vi "Fc_update_params_from_uc.vi"(7 "Class TCP":T1, 8 "error in (no error)":errorcluster, 9 "Trace names":refnum<vi>, 10 "# Control":refnum<vi>, 11 "SamplesXSignal?":refnum<vi>) -> (0 "error out":errorcluster, 1 "TRACE_SIZE":i32, 2 "NB_TRACED_SIGNALS":i32, 3 "CS STATUS":i32)   [LabVIEW 2022 SP3]
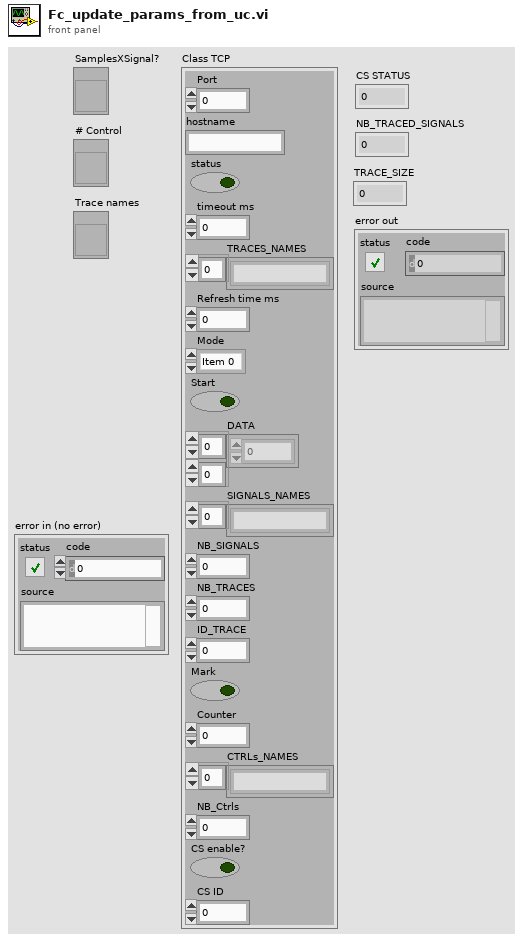
[diagram p1: front panel]
types:
  T1 = cluster{"Port":i32, "hostname":string, "status":bool, "timeout ms":i32, "TRACES_NAMES":string[], "Refresh time ms":i32, "Mode":enum32{"Item 0", "Item 1"}, "Start":bool, "DATA":sgl[][], "SIGNALS_NAMES":string[], "NB_SIGNALS":i32, "NB_TRACES":i32, "ID_TRACE":i32, "Mark":bool, "Counter":i32, "CTRLs_NAMES":string[], "NB_Ctrls":i32, "CS enable?":bool, "CS ID":i32}
  T2 = cluster{"TRACE_SIZE":i32, "CS_ID":i32, "TRACE ID":i32, "CMD":i32, "DATA(M)":i32}
  T3 = cluster{"timeout ms":i32, "remote port":u16, "Address":string}
  T4 = cluster{"SIZE":i32, " TRACE DATA":sgl[], "TRACE_SIZE":i32, "NB_TRACES":i32, "NB_TRACED_SIGNALS":i32, "NAMES TRACED SIGNALS":string[], "NAMES TRACES":string[], "CS STATUS":i32, "NB_CSs":i32, "NAMES CSs":string[], "DATA (M)":sgl[], "CMD":i32}
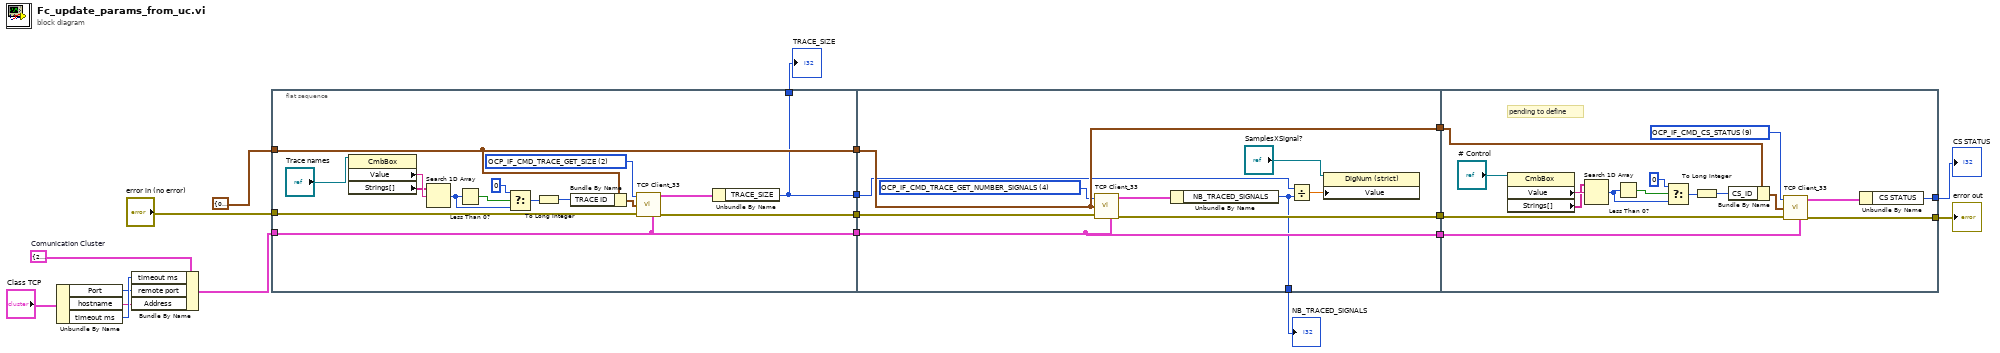
[diagram p0: block diagram]
diagram:
  w12 = T3 {"timeout ms"=2000, "remote port"=8085, "Address"="127.0.0.1"}  # Comunication Cluster
  n1 = Unbundle By Name("Class TCP") -> ("Port"=w3:i32, "hostname"=w4:string, "timeout ms"=w5:i32)
  n2 = Bundle By Name(cluster=w12, "timeout ms"=w5, "remote port"=w3, "Address"=w4) -> (w6:T3)
  n3 = flat-sequence {
    tunnel: T2 {"TRACE_SIZE"=0, "CS_ID"=0, "TRACE ID"=0, "CMD"=0, "DATA(M)"=0} ("Input Cluster") -> [w32]
    tunnel: [w32] -> w19
    tunnel: [w34] -> w18
    tunnel: w6 -> [w33]
    tunnel: [w33] -> w17
    tunnel: [w24] -> w16
    tunnel: [w24] -> w9
    tunnel: "error in (no error)" -> [w20]
    tunnel: w19 -> [w43]
    tunnel: [w43] -> w15
    tunnel: w18 -> [w45]
    tunnel: [w44] -> w14
    tunnel: w17 -> [w42]
    tunnel: [w42] -> w13
    tunnel: w16 -> [w39]
    tunnel: [w38] -> w10
    tunnel: [w57] -> w2
    tunnel: w15 -> [w60]
    tunnel: w14 -> [w56]
    tunnel: w13 -> [w55]
    tunnel: [w49] -> w11
    frame #0 {
      w35 = 2 items=["OCP_IF_CMD_TRACE_READ", "OCP_IF_CMD_TRACE_RESET", "OCP_IF_CMD_TRACE_GET_SIZE", "OCP_IF_CMD_TRACE_SET_SIZE", "OCP_IF_CMD_TRACE_GET_NUMBER_SIGNALS", "OCP_IF_CMD_TRACE_GET_SIGNALS_NAMES", "OCP_IF_CMD_TRACE_GET_NUMBER_TRACES", "OCP_IF_CMD_TRACE_GET_TRACES_NAMES", "OCP_IF_CMD_TRACE_GET_ADDRESS", "OCP_IF_CMD_CS_STATUS", "OCP_IF_CMD_CS_ENABLE", "OCP_IF_CMD_CS_DISABLE", "OCP_IF_CMD_CS_CONTROLLER_IF", "OCP_IF_CMD_CS_HARDWARE_IF", "OCP_IF_CMD_CS_GET_NUMBER_CONTROLLERS", "OCP_IF_CMD_CS_GET_CONTROLLERS_NAMES", "OCP_IF_CMD_PLATFORM_ID", "OCP_IF_CMD_PLATFORM_IF", "OCP_IF_CMD_OPIL_UPDATE_MEASUREMENTS", "OCP_IF_CMD_OPIL_UPDATE_SIM_DATA", "OCP_IF_CMD_OPIL_RUN_CONTROL", "OCP_IF_CMD_OPIL_INITIALIZE_CONTROL", "OCP_IF_CMD_OPIL_GET_CONTROL", "OCP_IF_CMD_OPIL_GET_CONTROLLER_DATA", "OCP_IF_CMD_END"] ("CMD")
      n4 = property class="CmbBox"(reference="Trace names") -> ("Value"=w23:string, "Strings[]"=w22:string[])  [unwired: 1 in, 2 out]
      n5 = Search 1D Array(1D array=w22, element=w23) -> (index of element=w26:i32)  [unwired: 1 in]
      n6 = Less Than 0?(x=w26) -> (x < 0?=w27:bool)
      n7 = Select(t=0, s=w27, f=w26) -> (s? t:f=w25:i32)
      n8 = To Long Integer(number=w25) -> (32bit integer=w29:i32)
      n9 = Bundle By Name(cluster=w32, "TRACE ID"=w29) -> (w31:T2)
      n10 = call "TCP Client_33.vi"("CMD"=w35, "Input Cluster"=w31, "error in (no error)"=w20, "Comunication Cluster"=w33) -> ("Output cluster"=w30:T4, "error out"=w34:errorcluster)  [unwired: 4 in, 1 out]
      n11 = Unbundle By Name(w30) -> ("TRACE_SIZE"=w24:i32)
    }
    frame #1 {
      w41 = 4 items=["OCP_IF_CMD_TRACE_READ", "OCP_IF_CMD_TRACE_RESET", "OCP_IF_CMD_TRACE_GET_SIZE", "OCP_IF_CMD_TRACE_SET_SIZE", "OCP_IF_CMD_TRACE_GET_NUMBER_SIGNALS", "OCP_IF_CMD_TRACE_GET_SIGNALS_NAMES", "OCP_IF_CMD_TRACE_GET_NUMBER_TRACES", "OCP_IF_CMD_TRACE_GET_TRACES_NAMES", "OCP_IF_CMD_TRACE_GET_ADDRESS", "OCP_IF_CMD_CS_STATUS", "OCP_IF_CMD_CS_ENABLE", "OCP_IF_CMD_CS_DISABLE", "OCP_IF_CMD_CS_CONTROLLER_IF", "OCP_IF_CMD_CS_HARDWARE_IF", "OCP_IF_CMD_CS_GET_NUMBER_CONTROLLERS", "OCP_IF_CMD_CS_GET_CONTROLLERS_NAMES", "OCP_IF_CMD_PLATFORM_ID", "OCP_IF_CMD_PLATFORM_IF", "OCP_IF_CMD_OPIL_UPDATE_MEASUREMENTS", "OCP_IF_CMD_OPIL_UPDATE_SIM_DATA", "OCP_IF_CMD_OPIL_RUN_CONTROL", "OCP_IF_CMD_OPIL_INITIALIZE_CONTROL", "OCP_IF_CMD_OPIL_GET_CONTROL", "OCP_IF_CMD_OPIL_GET_CONTROLLER_DATA", "OCP_IF_CMD_END"] ("CMD")
      n12 = call "TCP Client_33.vi"("CMD"=w41, "Input Cluster"=w43, "error in (no error)"=w45, "Comunication Cluster"=w42) -> ("Output cluster"=w40:T4, "error out"=w44:errorcluster)  [unwired: 4 in, 1 out]
      n13 = Unbundle By Name(w40) -> ("NB_TRACED_SIGNALS"=w38:i32)
      n14 = Divide(x=w39, y=w38) -> (x/y=w37:dbl)
      n15 = property class="DigNum (strict)"(reference="SamplesXSignal?", "Value"=w37) -> ()  [unwired: 1 in, 2 out]
    }
    frame #2 {
      w59 = 9 items=["OCP_IF_CMD_TRACE_READ", "OCP_IF_CMD_TRACE_RESET", "OCP_IF_CMD_TRACE_GET_SIZE", "OCP_IF_CMD_TRACE_SET_SIZE", "OCP_IF_CMD_TRACE_GET_NUMBER_SIGNALS", "OCP_IF_CMD_TRACE_GET_SIGNALS_NAMES", "OCP_IF_CMD_TRACE_GET_NUMBER_TRACES", "OCP_IF_CMD_TRACE_GET_TRACES_NAMES", "OCP_IF_CMD_TRACE_GET_ADDRESS", "OCP_IF_CMD_CS_STATUS", "OCP_IF_CMD_CS_ENABLE", "OCP_IF_CMD_CS_DISABLE", "OCP_IF_CMD_CS_CONTROLLER_IF", "OCP_IF_CMD_CS_HARDWARE_IF", "OCP_IF_CMD_CS_GET_NUMBER_CONTROLLERS", "OCP_IF_CMD_CS_GET_CONTROLLERS_NAMES", "OCP_IF_CMD_PLATFORM_ID", "OCP_IF_CMD_PLATFORM_IF", "OCP_IF_CMD_OPIL_UPDATE_MEASUREMENTS", "OCP_IF_CMD_OPIL_UPDATE_SIM_DATA", "OCP_IF_CMD_OPIL_RUN_CONTROL", "OCP_IF_CMD_OPIL_INITIALIZE_CONTROL", "OCP_IF_CMD_OPIL_GET_CONTROL", "OCP_IF_CMD_OPIL_GET_CONTROLLER_DATA", "OCP_IF_CMD_END"] ("CMD")
      # "pending to define"
      n16 = property class="CmbBox"(reference="# Control") -> ("Value"=w48:string, "Strings[]"=w47:string[])  [unwired: 1 in, 2 out]
      n17 = Search 1D Array(1D array=w47, element=w48) -> (index of element=w52:i32)  [unwired: 1 in]
      n18 = Less Than 0?(x=w52) -> (x < 0?=w54:bool)
      n19 = Select(t=0, s=w54, f=w52) -> (s? t:f=w51:i32)
      n20 = To Long Integer(number=w51) -> (32bit integer=w50:i32)
      n21 = Bundle By Name(cluster=w60, "CS_ID"=w50) -> (w58:T2)
      n22 = call "TCP Client_33.vi"("CMD"=w59, "Input Cluster"=w58, "error in (no error)"=w56, "Comunication Cluster"=w55) -> ("Output cluster"=w61:T4, "error out"=w57:errorcluster)  [unwired: 4 in, 1 out]
      n23 = Unbundle By Name(w61) -> ("CS STATUS"=w49:i32)
    }
  }
  "CS STATUS" <- w11
  "NB_TRACED_SIGNALS" <- w10
  "TRACE_SIZE" <- w9
  "error out" <- w2
